vi "Connection State Callback.vi"(7 "Owner":refnum<class>, 8 "error in (no error)":errorcluster, 10 "Connection State":T1, 11 "Connection":refnum<class "Connection.lvclass">) -> (0 "error out":errorcluster)   [LabVIEW 2020, in "Stream-Simple-Msg.lvlib" / "Manager.lvclass"]
uses:
  Manager.lvclass
  lv-stream/stream/Connection/Connection.lvclass
  lv-stream/stream/Connection State.ctl
  lv-stream/stream/Stream.lvlib
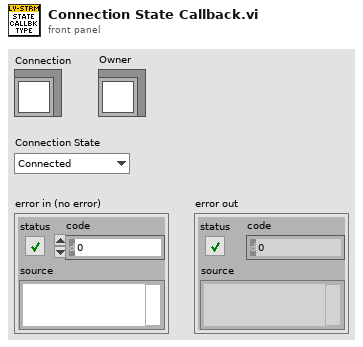
[diagram p1: front panel]
types:
  T1 = typedef "Stream.lvlib/Connection State.ctl" = enum16{"Connected", "Disconnected"}
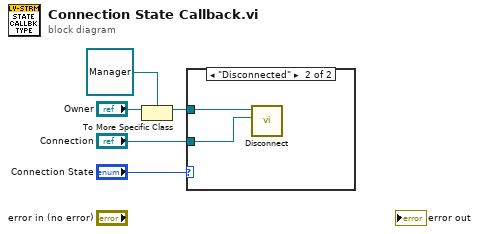
[diagram p0: block diagram]
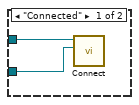
[diagram p2: hidden frame]
diagram:
  n1 = To More Specific Class(target class=refnum<class "Manager.lvclass"> refnum ("Stream-Simple-Msg:Manager"), reference="Owner") -> (specific class reference=w2:refnum<class "Manager.lvclass">)  [unwired: 1 in, 1 out]
  n2 = case shown="\"Disconnected\"" "Connection State" {
    tunnel: w2 -> [w7 w9]
    tunnel: "Connection" -> [w6 w8]
    frame "Connected" {
      n3 = call "Connect.vi"("Stream:Connection"=w6, "Manager in"=w7) -> ()  [unwired: 8 in, 2 out]
    }
    frame "Disconnected" {
      n4 = call "Disconnect.vi"("Stream:Connection"=w8, "Manager in"=w9) -> ()  [unwired: 8 in, 2 out]
    }
  }
